vi "_ROSMasterConsole.vi"() -> ()   [LabVIEW 2013]
uses:
  <vilib>/Utility/miscctls.llb/LVRectTypeDef.ctl
  _ROSDefinition.vi
panel:
  in  "Clear Servers?":bool
  in  "expand?":bool
  out "Status":string
  out "Master?":bool
  in  "Tab Control":enum32{"Single Calls", "Servers"}(tab)
  out "TCP Calls":T1(array[cluster])
  out "ROS Master":string="192.168.1.110:11311"
  out "Running?":bool
  out "current task":string
  in  "Stop":bool
  in  "Live Servers":i32(listbox)
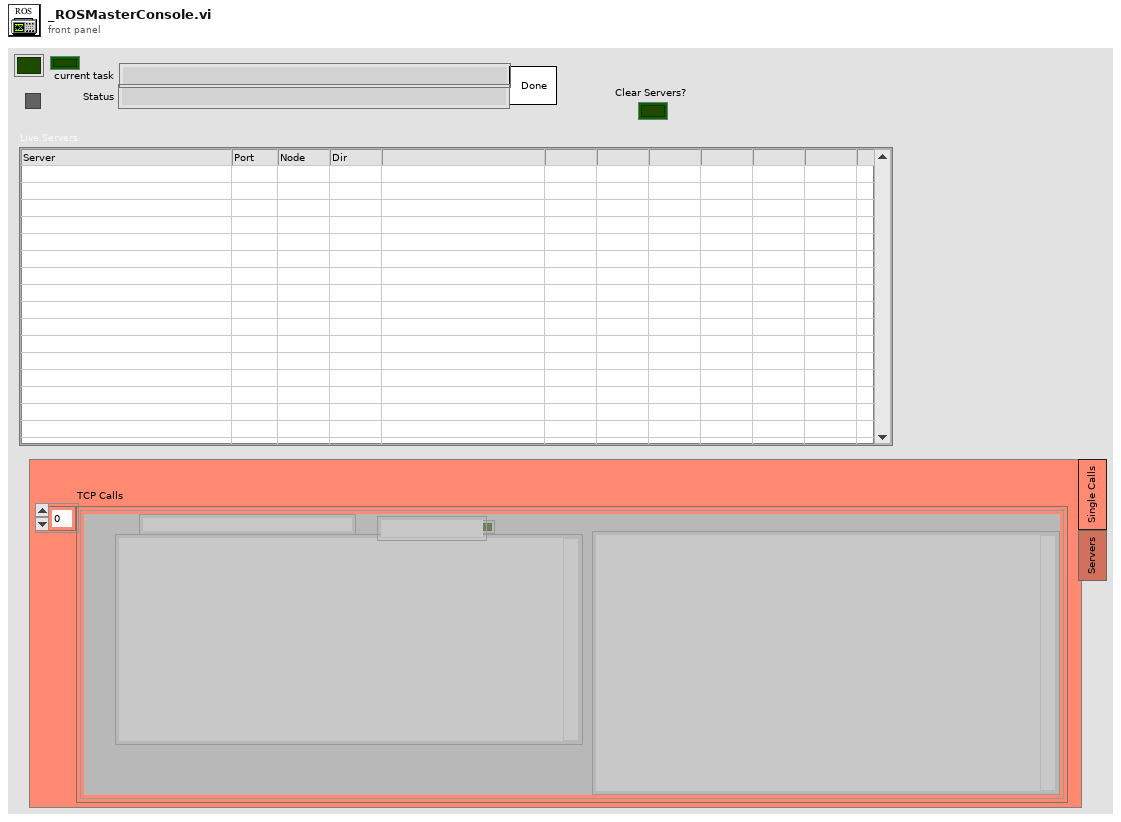
[diagram p1: front panel]
types:
  T1 = cluster{"First":string, "Second":string, "MethodName":string, "success":bool, "Dir1":string, "Dir2":string, "time":string}[]
  T2 = cluster{"server vi":string, "reference":refnum<vi>, "Description":string[], bool}[]
  T3 = cluster{"data out":string, "data out 2":string, "data out 3":string, "Success?":bool, "data out 4":string, "data out 5":string, "time":string}[]
  T4 = cluster{"Request":string, "Reply":string, "MethodName":string, "success":bool, "first string":string, "second string":string, "second string 2":string}
  T5 = typedef "LVRectTypeDef.ctl" = cluster{"Left":i16, "Top":i16, "Right":i16, "Bottom":i16}
  T6 = cluster{"server vi":string, "reference":refnum<vi>, "Description":string[], "Connected":bool}[]
  T7 = typedef "_ROSControl.ctl" = cluster{"topic port":u16, "Node":string, "topic":string, "type":string, "node port":u32, "error ":errorcluster, "Direction":T8, "APIs":string[]}
  T8 = typedef "_ROSDirection.ctl" = enum16{"Node", "Publisher", "Subscriber", "Service Client"}
  T9 = cluster{"server vi":string, "reference":refnum<vi>, "Description":string[], "Connected":bool}
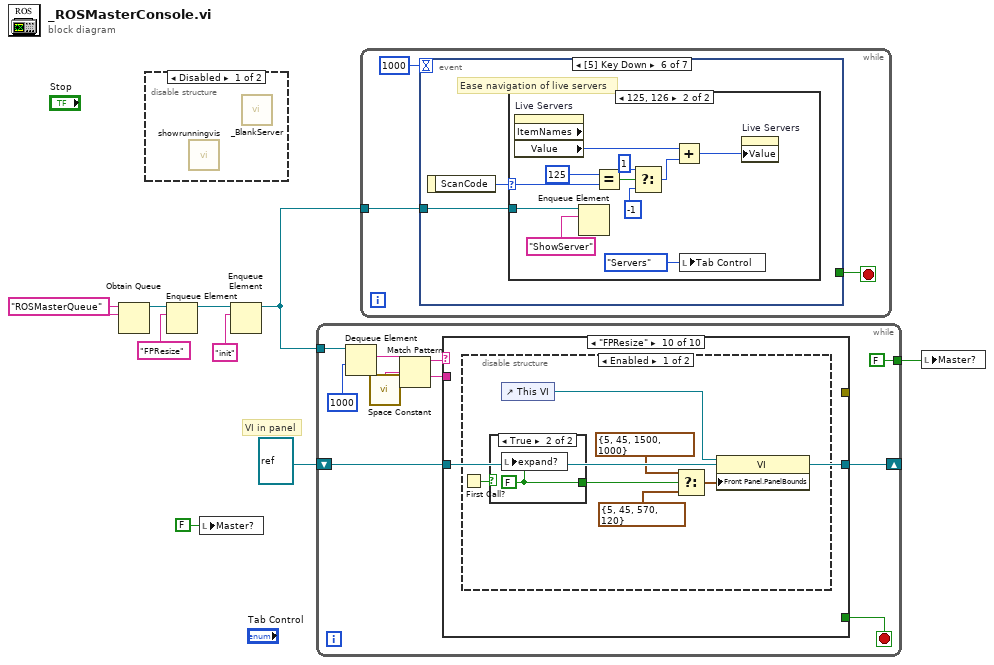
[diagram p0: block diagram]
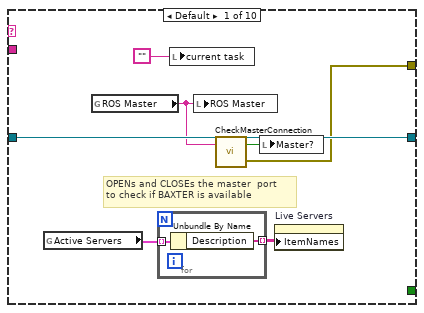
[diagram p3: hidden frame]
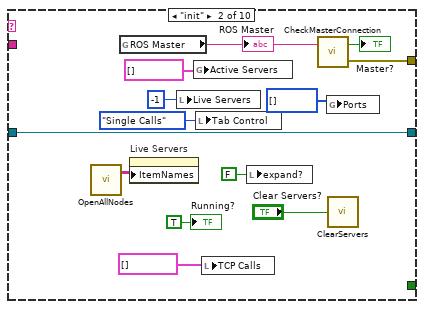
[diagram p4: hidden frame]
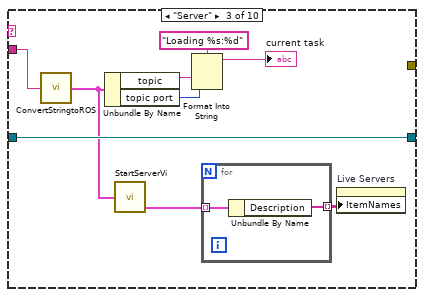
[diagram p5: hidden frame]
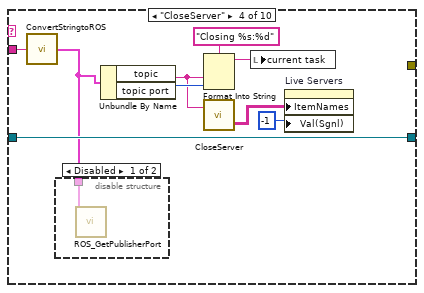
[diagram p6: hidden frame]
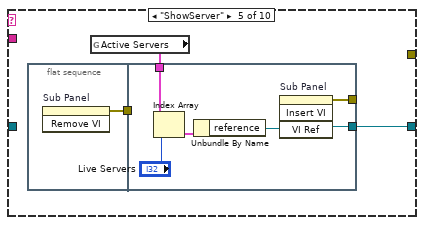
[diagram p8: hidden frame]
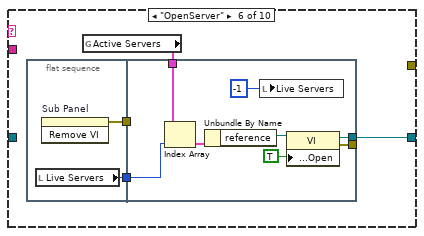
[diagram p9: hidden frame]
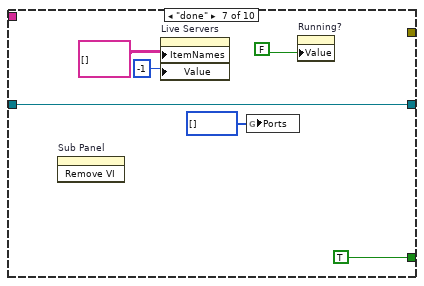
[diagram p10: hidden frame]
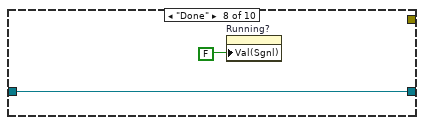
[diagram p11: hidden frame]
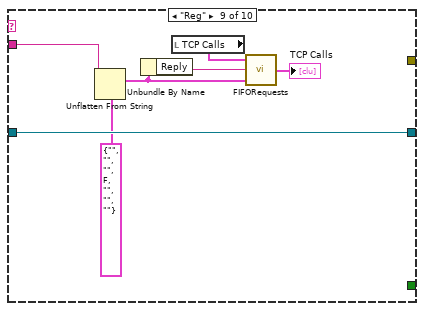
[diagram p12: hidden frame]
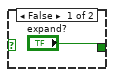
[diagram p13: hidden frame]
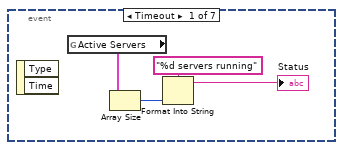
[diagram p15: hidden frame]
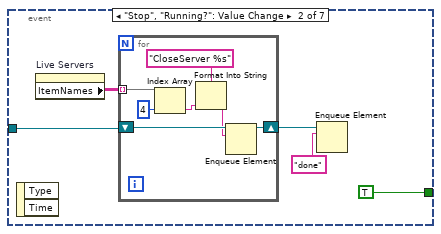
[diagram p16: hidden frame]
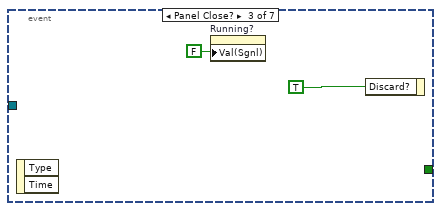
[diagram p17: hidden frame]
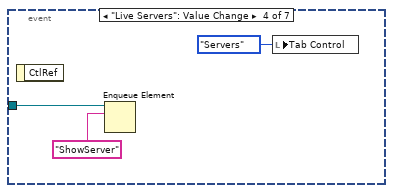
[diagram p18: hidden frame]
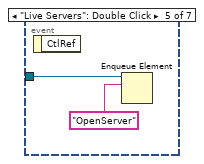
[diagram p19: hidden frame]
diagram:
  w9 = "ROSMasterQueue" ("name (unnamed)")
  # "VI in panel"
  n1 = Obtain Queue(name (unnamed)=w9, element data type=w9) -> (queue out=w6:refnum<queue>)  [unwired: 3 in, 2 out]
  n2 = disable-structure shown="Disabled" {
    frame Disabled {
      n3 = call "showrunningvis.vi"() -> ()  [unwired: 1 in]
      n4 = call "_BlankServer.vi"() -> ()  [unwired: 12 in]
    }
    frame Enabled {
    }
  }
  n5 = Enqueue Element(queue=w6, element="FPResize") -> (queue out=w5:refnum<queue>)  [unwired: 2 in, 2 out]
  n6 = local write "Master?"(FALSE ("Master?")) -> ()
  n7 = Enqueue Element(queue=w5, element="init") -> (queue out=w8:refnum<queue>)  [unwired: 2 in, 2 out]
  n8 = while {
    tunnel: w8 -> [w19]
    shift-right: [w12] -> _
    shift-left: refnum<vi> refnum ("VI Ref") -> [w13]
    tunnel: [FALSE] -> w1
    stop <- w18 stop-if-true
    n9 = Dequeue Element(queue=w19, timeout in ms (-1)=1000) -> (element=w16:string)  [unwired: 1 in, 3 out]
    n10 = call <vilib>:"Space Constant.vi"() -> ("String"=w15:string)
    n11 = Match Pattern(string=w16, regular expression=w15) -> (before substring=w17:string, after substring=w14:string)  [unwired: 1 in, 2 out]
    n12 = case shown="\"FPResize\"" w17 {
      tunnel: [_ _ _ _ _ _ TRUE _ _ _] -> w18
      tunnel: w14 -> [_ _ w47 w56 _ _ _ _ w99 _]
      tunnel: w13 -> [w26 w41 w50 w61 _ _ w90 w93 w100 w101]
      tunnel: [w26 w41 w50 w61 w63 w72 w90 w93 w100 w101] -> w12
      tunnel: [w22 w29 _ _ _ _ _ _ _ _] -> _
      frame Default {
        # "OPENs and CLOSEs the master  port\nto check if BAXTER is available"
        n13 = global read "_ROSDefinition.vi" "Active Servers"() -> (w21:T6)
        n14 = global read "_ROSDefinition.vi" "ROS Master"() -> (w24:string)
        n15 = for {
          tunnel: w21 -> [w28] mode=indexing
          tunnel: [w27] -> w20 mode=indexing
          n16 = Unbundle By Name(w28) -> ("Description"=w27:string[])
        }
        n17 = local write "current task"("") -> ()
        n18 = local write "ROS Master"(w24) -> ()
        n19 = call "CheckMasterConnection.vi"("Master IP"=w24) -> ("error out"=w22:errorcluster, "Master There?"=w23:bool)  [unwired: 1 in]
        n20 = local write "Master?"(w23) -> ()
        n21 = property on="Live Servers" class="MCListbox (strict)"("ItemNames"=w20) -> ()  [unwired: 2 in, 2 out]
      }
      frame "init" {
        n22 = call "OpenAllNodes.vi"() -> ("Nodes"=w39:string[][])  [unwired: 2 in]
        n23 = global read "_ROSDefinition.vi" "ROS Master"() -> (w31:string)
        "ROS Master" <- w31
        n24 = property on="Live Servers" class="MCListbox (strict)"("ItemNames"=w39) -> ()  [unwired: 2 in, 2 out]
        n25 = local write "Live Servers"(-1 ("Live Servers")) -> ()
        n26 = global write "_ROSDefinition.vi" "Active Servers"(T2 [] ("Active Servers")) -> ()
        n27 = local write "Tab Control"(enum32{"Single Calls", "Servers"}."Single Calls" ("Tab Control")) -> ()
        n28 = local write "TCP Calls"(T3 [] ("TCP Calls")) -> ()
        n29 = local write "expand?"(FALSE ("expand?")) -> ()
        n30 = call "CheckMasterConnection.vi"("Master IP"=w31) -> ("error out"=w29:errorcluster, "Master There?"=→"Master?":bool)  [unwired: 1 in]
        n31 = global write "_ROSDefinition.vi" "Ports"(u16[] [] ("Ports")) -> ()
        n32 = call "ClearServers.vi"("Clear Servers?"="Clear Servers?") -> ()  [unwired: 1 out]
        "Running?" <- TRUE ("Running?")
      }
      frame "Server" {
        n33 = call "ConvertStringtoROS.vi"("string in"=w47) -> ("ROS"=w43:T7)
        n34 = Unbundle By Name(w43) -> ("topic"=w46:string, "topic port"=w45:u16)
        n35 = call "StartServerVi.vi"("Baxter"=w43) -> ("Active Topics"=w44:T6)  [unwired: 2 out]
        n36 = Format Into String(format string="Loading %s:%d", w46, w45) -> (resulting string=→"current task":string)  [unwired: 2 in, 1 out]
        n37 = for {
          tunnel: w44 -> [w52] mode=indexing
          tunnel: [w51] -> w42 mode=indexing
          n38 = Unbundle By Name(w52) -> ("Description"=w51:string[])
        }
        n39 = property on="Live Servers" class="MCListbox (strict)"("ItemNames"=w42) -> ()  [unwired: 2 in, 2 out]
      }
      frame "CloseServer" {
        n40 = call "ConvertStringtoROS.vi"("string in"=w56) -> ("ROS"=w53:T7)
        n41 = disable-structure shown="Disabled" {
          disable-tunnel: w53 -> [w62 _]
          frame Disabled {
            n42 = call "ROS_GetPublisherPort.vi"("ROS in"=w62) -> ()  [unwired: 1 in, 2 out]
          }
          frame Enabled {
          }
        }
        n43 = Unbundle By Name(w53) -> ("topic"=w54:string, "topic port"=w55:u16)
        n44 = Format Into String(format string="Closing %s:%d", w54, w55) -> (resulting string=w59:string)  [unwired: 2 in, 1 out]
        n45 = call "CloseServer.vi"("Server"=w54) -> ("Active Servers Out"=w58:string[][])  [unwired: 2 in]
        n46 = local write "current task"(w59) -> ()
        n47 = property on="Live Servers" class="MCListbox (strict)"("ItemNames"=w58, "Val(Sgnl)"=-1 ("Value (Signaling)")) -> ()  [unwired: 2 in, 2 out]
      }
      frame "ShowServer" {
        n48 = flat-sequence {
          tunnel: [w66] -> w65
          tunnel: w65 -> [_]
          tunnel: [w70] -> _
          tunnel: w64 -> [w69]
          tunnel: [w67] -> w63
          frame #0 {
            n49 = invoke on="Sub Panel" class="SubPanel" method="Remove VI"() -> (error out=w66:errorcluster)  [unwired: 3 in, 2 out]
          }
          frame #1 {
            n50 = Index Array(array=w69, index="Live Servers") -> (element=w68:T9)
            n51 = Unbundle By Name(w68) -> ("reference"=w67:refnum<vi>)
            n52 = invoke on="Sub Panel" class="SubPanel" method="Insert VI"("VI Ref"=w67) -> (error out=w70:errorcluster)  [unwired: 3 in, 3 out]
          }
        }
        n53 = global read "_ROSDefinition.vi" "Active Servers"() -> (w64:T6)
      }
      frame "OpenServer" {
        n54 = flat-sequence {
          tunnel: [w77] -> w75
          tunnel: [w76] -> w74
          tunnel: w75 -> [_]
          tunnel: w74 -> [w84]
          tunnel: w73 -> [w82]
          tunnel: [w79] -> w72
          tunnel: [w78] -> _
          frame #0 {
            n55 = local read "Live Servers"() -> (w76:i32)
            n56 = invoke on="Sub Panel" class="SubPanel" method="Remove VI"() -> (error out=w77:errorcluster)  [unwired: 3 in, 2 out]
          }
          frame #1 {
            n57 = Index Array(array=w82, index=w84) -> (element=w81:T9)
            n58 = Unbundle By Name(w81) -> ("reference"=w80:refnum<vi>)
            n59 = local write "Live Servers"(-1 ("Live Servers")) -> ()
            n60 = property class="VI"(reference=w80, "Front Panel.Open"=TRUE ("Front Panel Window:Open")) -> (reference out=w79:refnum<vi>, error out=w78:errorcluster)  [unwired: 1 in]
          }
        }
        n61 = global read "_ROSDefinition.vi" "Active Servers"() -> (w73:T6)
      }
      frame "done" {
        n62 = invoke on="Sub Panel" class="SubPanel" method="Remove VI"() -> ()  [unwired: 3 in, 3 out]
        n63 = property on="Live Servers" class="MCListbox (strict)"("ItemNames"=string[][] [] ("Item Names"), "Value"=-1 ("Live Servers")) -> ()  [unwired: 2 in, 2 out]
        n64 = global write "_ROSDefinition.vi" "Ports"(u16[] [] ("Ports")) -> ()
        n65 = property on="Running?" class="Bool (strict)"("Value"=FALSE) -> ()  [unwired: 2 in, 2 out]
      }
      frame "Done" {
        n66 = property on="Running?" class="Bool (strict)"("Val(Sgnl)"=FALSE) -> ()  [unwired: 2 in, 2 out]
      }
      frame "Reg" {
        n67 = Unflatten From String(type=T4 {"Request"="", "Reply"="", "MethodName"="", "success"=FALSE, "first string"="", "second string"="", "second string 2"=""} ("Reg"), binary string=w99) -> (value=w95:T4)  [unwired: 3 in, 2 out]
        n68 = Unbundle By Name(w95) -> ("Reply"=w94:string)
        n69 = local read "TCP Calls"() -> (w97:T1)
        n70 = call "FIFORequests.vi"("New One"=w95, "data out"=w94, "Requests In"=w97) -> ("Requests Out"=→"TCP Calls":T3)
      }
      frame "FPResize" {
        n71 = disable-structure shown="Enabled" {
          frame Enabled {
            n72 = First Call?() -> (First Call?: T/F=w103:bool)
            n73 = case shown="True" w103 {
              tunnel: ["expand?" w109] -> w102
              frame False {
              }
              frame True {
                w109 = FALSE ("expand?")
                n74 = local write "expand?"(w109) -> ()
              }
            }
            n75 = control-ref of="This VI"() -> (w107:refnum<vi>)
            n76 = Select(t=T5 {"Left"=5, "Top"=45, "Right"=1500, "Bottom"=1000} ("Front Panel Window:Panel Bounds"), s=w102, f=T5 {"Left"=5, "Top"=45, "Right"=570, "Bottom"=120} ("Front Panel Window:Panel Bounds")) -> (s? t:f=w105:T5)
            n77 = property class="VI"(reference=w107, "Front Panel.PanelBounds"=w105) -> ()  [unwired: 1 in, 2 out]
          }
          frame Disabled {
          }
        }
      }
    }
  }
  n78 = while {
    tunnel: w8 -> [w112]
    stop <- w111 stop-if-true
    n79 = event shown="[5] Key Down" {
      selector: _ -> [_ _ _ _ _ _ _]
      dyn-events: _ -> [_ _ _ _ _ _ _]
      timeout: 1000 -> [_ _ _ _ _ _ _]
      tunnel: w112 -> [_ w119 _ w132 w134 w137 w149]
      tunnel: [_ TRUE ("Stop") _ _ _ _ _] -> w111
      event Timeout {
        n80 = event-data() -> ()  [unwired: 1 in, 2 out]
        n81 = global read "_ROSDefinition.vi" "Active Servers"() -> (w113:T6)
        n82 = Array Size(array=w113) -> (size(s)=w116:i32)
        n83 = Format Into String(format string="%d servers running", w116) -> (resulting string=→"Status":string)  [unwired: 2 in, 1 out]
      }
      event "Stop", "Running?": Value Change {
        n84 = event-data() -> ()  [unwired: 1 in, 2 out]
        n85 = property on="Live Servers" class="MCListbox (strict)"() -> ("ItemNames"=w120:string[][])  [unwired: 2 in, 2 out]
        n86 = for {
          tunnel: w120 -> [w128] mode=indexing
          shift-right: [w122] -> w118
          shift-left: w119 -> [w124]
          n87 = Index Array(array=w128, index=4) -> (element=w126:string)
          n88 = Format Into String(format string="CloseServer %s", w126) -> (resulting string=w123:string)  [unwired: 2 in, 1 out]
          n89 = Enqueue Element(queue=w124, element=w123) -> (queue out=w122:refnum<queue>)  [unwired: 2 in, 2 out]
        }
        n90 = Enqueue Element(queue=w118, element="done") -> ()  [unwired: 2 in, 3 out]
      }
      event Panel Close? {
        n91 = event-data() -> ()  [unwired: 1 in, 2 out]
        n92 = property on="Running?" class="Bool (strict)"("Val(Sgnl)"=FALSE ("Value (Signaling)")) -> ()  [unwired: 2 in, 2 out]
        n93 = event-data("Discard?"=TRUE ("Stop")) -> ()  [unwired: 1 in, 1 out]
      }
      event "Live Servers": Value Change {
        n94 = event-data() -> ()  [unwired: 1 in, 1 out]
        n95 = Enqueue Element(queue=w132, element="ShowServer") -> ()  [unwired: 2 in, 3 out]
        n96 = local write "Tab Control"(enum32{"Single Calls", "Servers"}."Servers" ("Tab Control")) -> ()
      }
      event "Live Servers": Double Click {
        n97 = event-data() -> ()  [unwired: 1 in, 1 out]
        n98 = Enqueue Element(queue=w134, element="OpenServer") -> ()  [unwired: 2 in, 3 out]
      }
      event Key Down {
        # "Ease navigation of live servers"
        n99 = event-data() -> ("ScanCode"=w136:i16)  [unwired: 1 in]
        n100 = case shown="125, 126" w136 {
          selector: w136 -> [_ w145]
          tunnel: w137 -> [_ w148]
          frame Default {
          }
          frame 125, 126 {
            n101 = property on="Live Servers" class="MCListbox (strict)" props=["ItemNames", "Value"]() -> ("Value"=w142:i32)  [unwired: 2 in, 3 out]
            n102 = Enqueue Element(queue=w148, element="ShowServer") -> ()  [unwired: 2 in, 3 out]
            n103 = Equal?(x=i16 125, y=w145) -> (x = y?=w143:bool)
            n104 = Select(t=i16 1 ("x"), s=w143, f=i16 -1 ("x")) -> (s? t:f=w141:i16)
            n105 = Add(x=w142, y=w141) -> (x+y=w138:i32)
            n106 = local write "Tab Control"(enum32{"Single Calls", "Servers"}."Servers" ("Tab Control")) -> ()
            n107 = property on="Live Servers" class="MCListbox (strict)"("Value"=w138) -> ()  [unwired: 2 in, 2 out]
          }
        }
      }
      event "expand?": Value Change {
        n108 = event-data() -> ()  [unwired: 1 in, 3 out]
        n109 = Enqueue Element(queue=w149, element="FPResize") -> ()  [unwired: 2 in, 3 out]
      }
    }
  }
  n110 = local write "Master?"(w1) -> ()
